vi "Login.vi"() -> ()   [LabVIEW 2021]
uses:
  <vilib>/Utility/file.llb/Write Delimited Spreadsheet (string).vi
panel:
  in  "Table Control":string[][](table)
  out "Boolean":bool
  in  "DELETE":bool
  in  "LOGIN":bool
  in  "Add":bool
  in  "PASSWORD":string
  in  "USERNAME":string
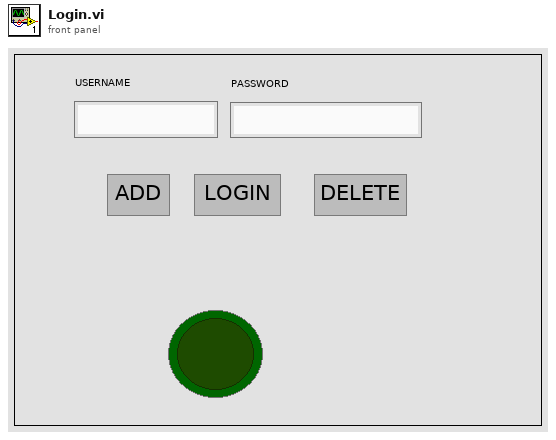
[diagram p1: front panel]
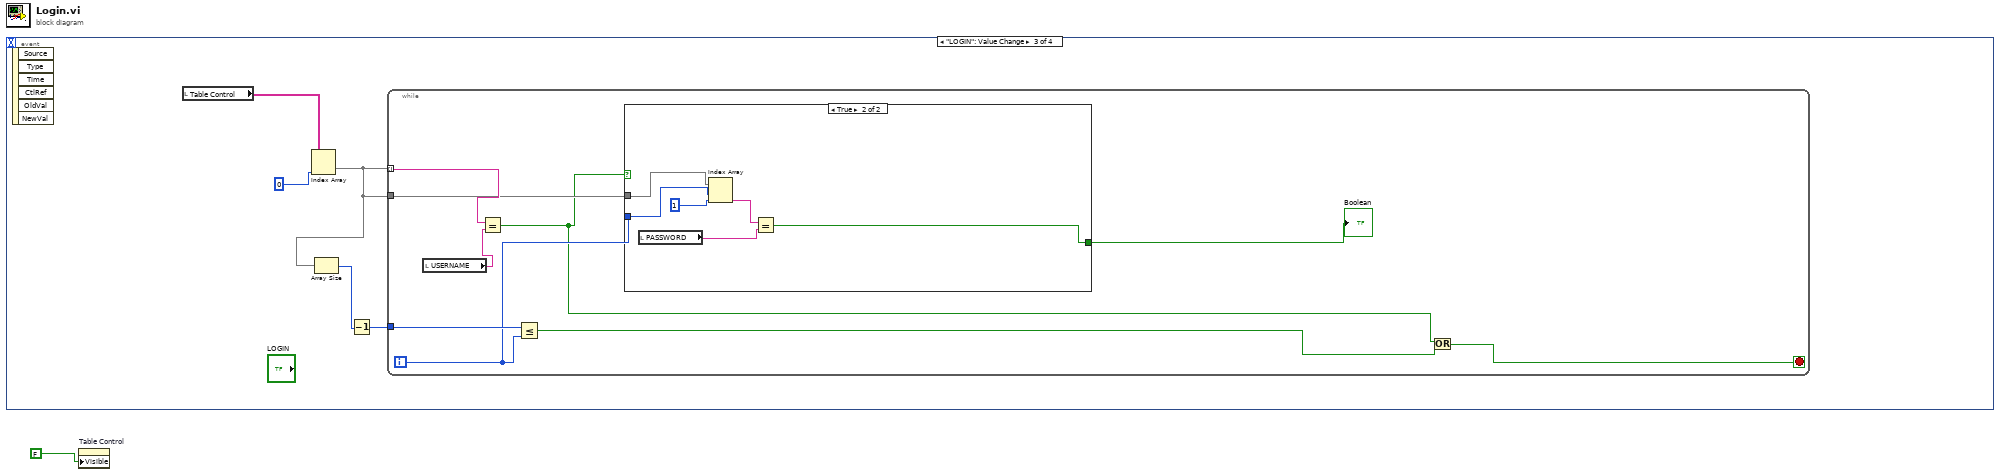
[diagram p0: block diagram]
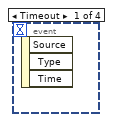
[diagram p2: hidden frame]
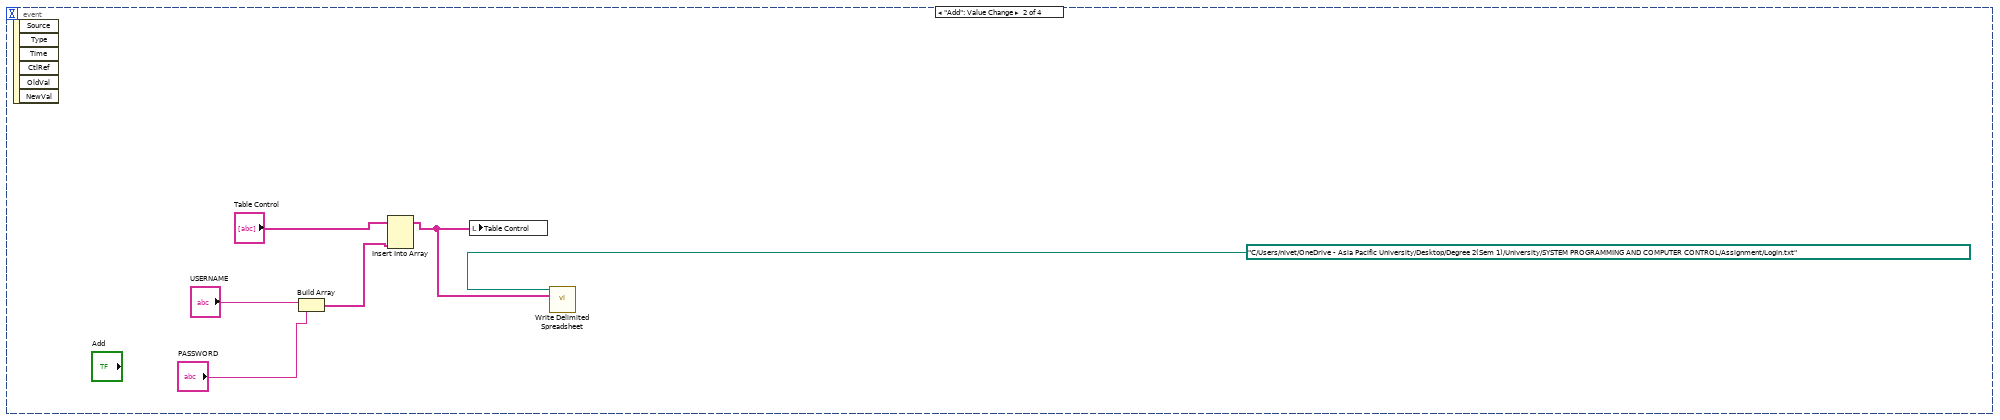
[diagram p3: hidden frame]
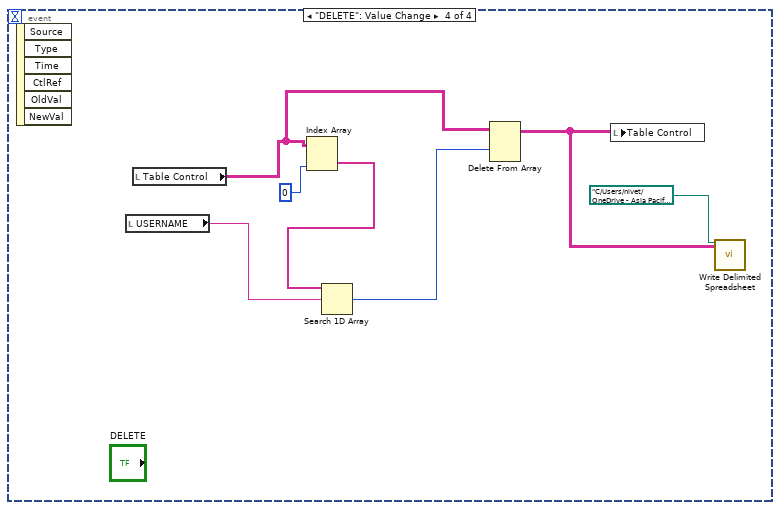
[diagram p5: hidden frame]
diagram:
  n1 = event shown="[2] \"LOGIN\": Value Change" {
    selector: _ -> [_ _ _ _]
    dyn-events: _ -> [_ _ _ _]
    timeout: _ -> [_ _ _ _]
    event Timeout {
      n2 = event-data() -> ()  [unwired: 1 in, 3 out]
    }
    event "Add": Value Change {
      n3 = event-data() -> ()  [unwired: 1 in, 6 out]
      n4 = Build Array "Build Array"("USERNAME", "PASSWORD") -> (w4:string[])
      n5 = Insert Into Array "Insert Into Array"(array="Table Control", new element=w4) -> (w3:string[][])  [unwired: 2 in]
      n6 = local write "Table Control"(w3) -> ()
      n7 = call-poly <vilib>:"Write Delimited Spreadsheet.vi"("file path (dialog if empty)"=path "C:/Users/nivet/OneDrive - Asia Pacific University/Desktop/Degree 2(Sem 1)/University/SYSTEM PROGRAMMING AND COMPUTER CONTROL/Assignment/Login.txt", "2D data"=w3) -> ()  [unwired: 12 in, 2 out]
    }
    event "LOGIN": Value Change {
      n8 = event-data() -> ()  [unwired: 1 in, 6 out]
      n9 = local read "Table Control"() -> (w12:string[][])
      n10 = Index Array "Index Array"(array=w12, index (col)=0) -> (element=w8:string[])  [unwired: 1 in]
      n11 = Array Size(array=w8) -> (size(s)=w10:i32)
      n12 = Decrement(x=w10) -> (x-1=w9:i32)
      n13 = while {
        tunnel: w8 -> [w20] mode=indexing
        tunnel: w9 -> [w19]
        tunnel: w8 -> [w17]
        i -> [w14]
        stop <- w16 stop-if-true
        n14 = local read "USERNAME"() -> (w21:string)
        n15 = Equal?(x=w20, y=w21) -> (x = y?=w13:bool)
        n16 = Less Or Equal?(x=w19, y=w14) -> (x <= y?=w18:bool)
        n17 = case shown="True" w13 {
          tunnel: [_ w23] -> w15
          tunnel: w17 -> [_ w25]
          tunnel: w14 -> [_ w22]
          frame False {
          }
          frame True {
            n18 = local read "PASSWORD"() -> (w24:string)
            n19 = Index Array "Index Array"(array=w25, index #1=w22, index #2=1) -> (element #2=w26:string)  [unwired: 1 out]
            n20 = Equal?(x=w26, y=w24) -> (x = y?=w23:bool)
          }
        }
        "Boolean" <- w15
        n21 = Or(x=w13, y=w18) -> (x .or. y?=w16:bool)
      }
    }
    event "DELETE": Value Change {
      n22 = event-data() -> ()  [unwired: 1 in, 6 out]
      n23 = local read "USERNAME"() -> (w34:string)
      n24 = local read "Table Control"() -> (w30:string[][])
      n25 = Index Array "Index Array"(array=w30, index (col)=0) -> (element=w32:string[])  [unwired: 1 in]
      n26 = Search 1D Array(1D array=w32, element=w34) -> (index of element=w31:i32)  [unwired: 1 in]
      n27 = Delete From Array "Delete From Array"(array=w30, index (row)=w31) -> (array with subset deleted=w29:string[][])  [unwired: 2 in, 1 out]
      n28 = local write "Table Control"(w29) -> ()
      n29 = call-poly <vilib>:"Write Delimited Spreadsheet.vi"("file path (dialog if empty)"=path "C:/Users/nivet/OneDrive - Asia Pacific University/Desktop/Degree 2(Sem 1)/University/SYSTEM PROGRAMMING AND COMPUTER CONTROL/Assignment/Login.txt", "2D data"=w29) -> ()  [unwired: 12 in, 2 out]
    }
  }
  n30 = property on="Table Control" class="Tbl (strict)"("Visible"=FALSE) -> ()  [unwired: 2 in, 2 out]
